vi "Rysuj Boidy.vi"(4 "color(black)":u32(colorbox), 6 "pen (Width 5)":T1={"Width"=5, "Style"=enum."Solid"}, 7 "Swiat in":picture, 8 "error in (no error)":errorcluster, 11 "Swiat in":refnum<class "Swiat.lvclass">) -> (0 "error out":errorcluster, 3 "Swiat out":refnum<class "Swiat.lvclass">, 5 "Swiat out":picture)   [LabVIEW 2014, in "Swiat.lvclass"]
uses:
  Swiat.lvclass
  Swiat.lvclass/Swiat.ctl
  Boid/Boid.lvclass/Boid.ctl
  Boid/Boid.lvclass
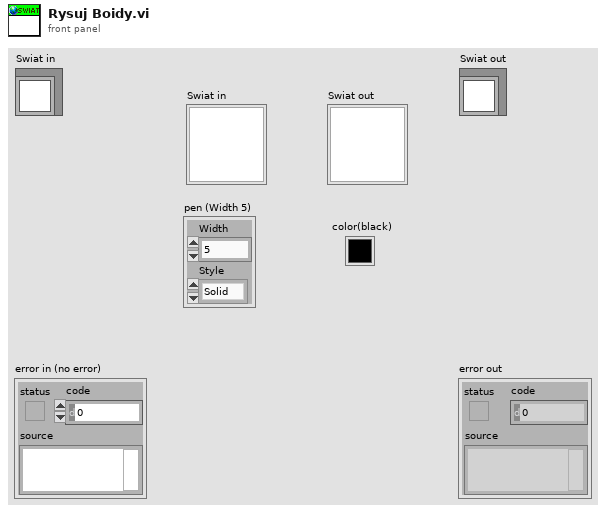
[diagram p1: front panel]
types:
  T1 = cluster{"Width":u16, "Style":enum32{"Solid", "Dash", "Dot", "DashDot", "DashDotDot"}}
  T2 = typedef "Position.ctl" = cluster{"x":i16, "y":i16}
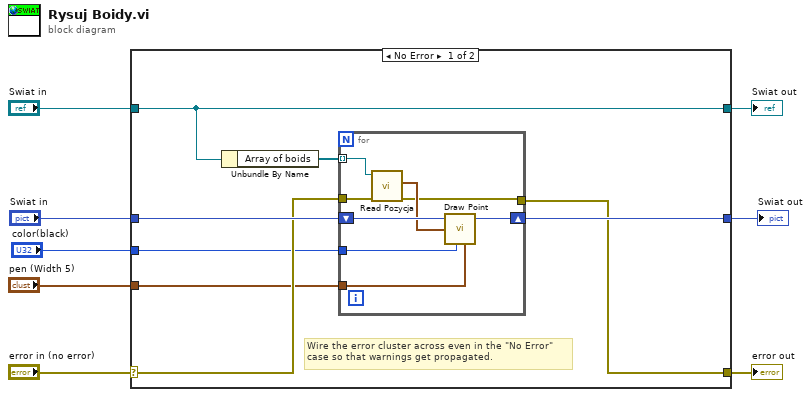
[diagram p0: block diagram]
diagram:
  n1 = case shown="No Error" "error in (no error)" {
    selector: "error in (no error)" -> [w12 w27]
    tunnel: [w11 w27] -> w7
    tunnel: [w16 w26] -> w5
    tunnel: "Swiat in" -> [w16 w26]
    tunnel: "Swiat in" -> [w14 w25]
    tunnel: [w13 w25] -> w3
    tunnel: "pen (Width 5)" -> [w10 _]
    tunnel: "color(black)" -> [w9 _]
    frame No Error {
      # "Wire the error cluster across even in the \"No Error\"\ncase so that warnings get propagated."
      n2 = Unbundle By Name(w16) -> ("Array of boids"=w15:refnum<class "Boid.lvclass">[])
      n3 = for {
        tunnel: w15 -> [w22] mode=indexing
        shift-right: [w23] -> w13
        shift-left: w14 -> [w24]
        tunnel: w12 -> [w20]
        tunnel: [w19] -> w11
        tunnel: w10 -> [w18]
        tunnel: w9 -> [w17]
        n4 = call "Read Pozycja.vi"("error in (no error)"=w20, "Boid in"=w22) -> ("error out"=w19:errorcluster, "Position"=w21:T2)  [unwired: 7 in, 1 out]
        n5 = call <vilib>:"Draw Point.vi"("picture"=w24, "point(x,y)"=w21, "color(black)"=w17, "pen"=w18) -> ("new picture"=w23:picture)  [unwired: 5 in]
      }
    }
    frame Error {
    }
  }
  "error out" <- w7
  "Swiat out" <- w5
  "Swiat out" <- w3
